vi "onDependencyStarted.vi"(8 "error in":errorcluster, 9 "Dependency":refnum<class "SMO.lvclass">, 11 "SMO in":refnum<class "SMO.lvclass">) -> (0 "error out":errorcluster, 3 "SMO out":refnum<class "SMO.lvclass">)   [LabVIEW 2013, in "SMO.lvclass"]
uses:
  SMO.lvclass
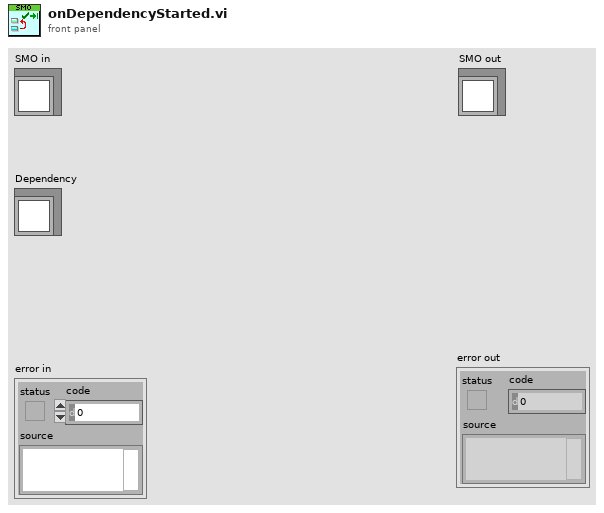
[diagram p1: front panel]
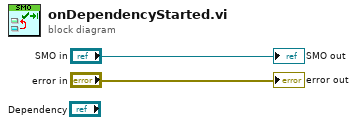
[diagram p0: block diagram]
diagram:
  "SMO out" <- "SMO in"
  "error out" <- "error in"
